vi "GenerateTargetList.vi"(11 "Detected Targets":T1[](array[typedef])) -> (3 "TargetList":string[](array[string]))   [LabVIEW 2021, in "myRIOMetaDataObj.lvclass"]
uses:
  myRIOMetaDataObj.lvclass
  <resource>/myRIO/Target Info.ctl
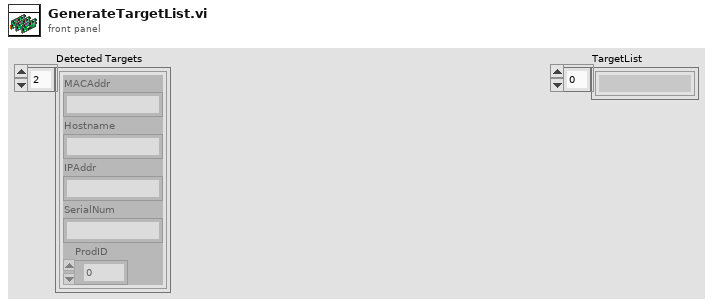
[diagram p1: front panel]
types:
  T1 = typedef "Target Info.ctl" = cluster{"MACAddr":string, "Hostname":string, "IPAddr":string, "SerialNum":string, "ProdID":u32}
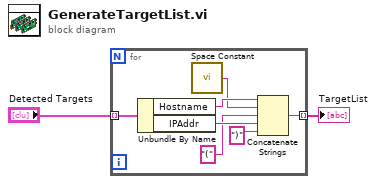
[diagram p0: block diagram]
diagram:
  n1 = for {
    tunnel: "Detected Targets" -> [w9] mode=indexing
    tunnel: [w5] -> w1 mode=indexing
    n2 = Unbundle By Name(w9) -> ("Hostname"=w4:string, "IPAddr"=w8:string)
    n3 = call <vilib>:"Space Constant.vi"() -> ("String"=w3:string)
    n4 = Concatenate Strings(w4, w3, "(" ("string"), w8, ")" ("string")) -> (w5:string)
  }
  "TargetList" <- w1
